vi "Request Synchronous Variant.vi"(6 "Ignore Past Updates? (F)":bool, 7 "Timeout In ms (-1)":i32=-1, 8 "error in (no error)":errorcluster, 9 "Type":variant, 10 "Datum Name":string, 11 "IObserver In":refnum<class "IObserver.lvclass">) -> (0 "error out":errorcluster, 1 "timed out?":bool, 2 "Data":variant, 4 "Publication Time":timestamp)   [LabVIEW 2020, in "IObserver.lvlib" / "IObserver.lvclass"]
doc: "DEPRECATED by Request Synchronous Data.vim"
uses:
  <vilib>/gpm_packages/@cs/mva-core/Source/IObserver/IObserver/IObserver.lvclass
  <vilib>/gpm_packages/@cs/mva-core/Source/IObserver/IObserver/IObserver.lvclass/IObserver.ctl
  <vilib>/gpm_packages/@cs/mva-core/Source/SubscriptionPolicy/OneShotSubscription/OneShotSubscription.lvclass/OneShotSubscription.ctl
  <vilib>/gpm_packages/@cs/transport/Source/Concrete/NotifierTransport/NotifierTransport.lvclass/NotifierTransport.ctl
  <vilib>/gpm_packages/@cs/mva-core/Source/IMediator/SubscriptionRequest/SubscriptionRequest.lvclass/SubscriptionRequest.ctl
  <vilib>/gpm_packages/@cs/mva-core/Source/IMediator/IMediator Messages/Subscribe Msg/Subscribe Msg.lvclass/Subscribe Msg.ctl
  <vilib>/gpm_packages/@cs/actor-framework-messages/Source/RoundTripMessage/RoundTripMessage.lvclass/RoundTripMessage.ctl
  <vilib>/ActorFramework/Message Enqueuer/Message Enqueuer.lvclass/Message Enqueuer.ctl
  <vilib>/gpm_packages/@cs/actor-framework-messages/Source/RoundTripMessage/Return Round-Trip Message.vi
  <vilib>/ActorFramework/Message Enqueuer/Enqueue.vi
  <vilib>/gpm_packages/@cs/transport/Source/Concrete/NotifierTransport/NotifierTransport.lvclass
  C:/Program Files/National Instruments/LabVIEW 2020/vi.lib/gpm_packages/@cs/transport/Source/ITransport/ITransport.lvclass
  <vilib>/gpm_packages/@cs/mva-core/Source/SubscriptionPolicy/OneShotSubscription/OneShotSubscription.lvclass
  C:/Program Files/National Instruments/LabVIEW 2020/vi.lib/gpm_packages/@cs/mva-core/Source/IMediator/ISubscriptionPolicy/ISubscriptionPolicy.lvclass
  <vilib>/gpm_packages/@cs/mva-core/Source/IMediator/IMediator Messages/Subscribe Msg/Subscribe Msg.lvclass
  C:/Program Files/National Instruments/LabVIEW 2020/vi.lib/gpm_packages/@cs/actor-framework-messages/Source/RoundTripMessage/RoundTripMessage.lvclass
  <vilib>/gpm_packages/@cs/actor-framework-messages/Source/RoundTripMessage/RoundTripMessage.lvclass
  C:/Program Files/National Instruments/LabVIEW 2020/vi.lib/ActorFramework/Message/Message.lvclass
  <vilib>/Utility/error.llb/Error Cluster From Error Code.vi
  <vilib>/ActorFramework/Message Priority Queue/Priority Enqueue.vi
  <vilib>/gpm_packages/@cs/mva-core/Source/IMediator/SubscriptionRequest/SubscriptionRequest.lvclass
  <vilib>/gpm_packages/@cs/mva-core/Source/IMediator/ISubscriptionPolicy/ISubscriptionPolicy.lvclass
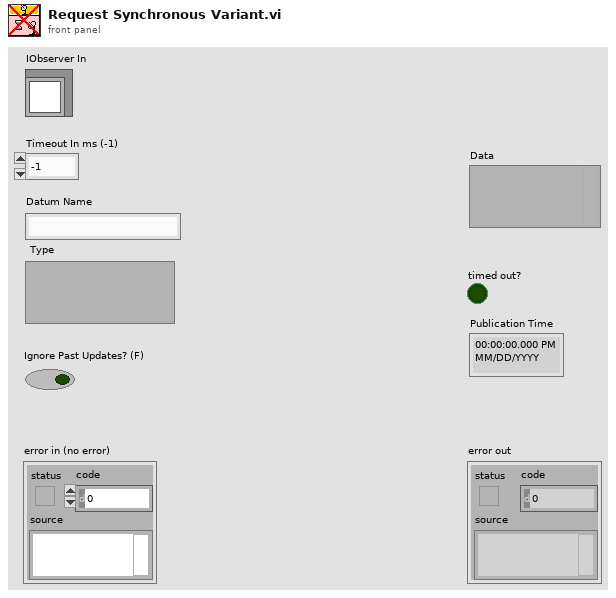
[diagram p1: front panel]
types:
  T1 = typedef "IMediator.lvlib/ISubscriptionPolicy.lvclass/ISubscriptionPolicy Reference.ctl" = refnum<data-value>
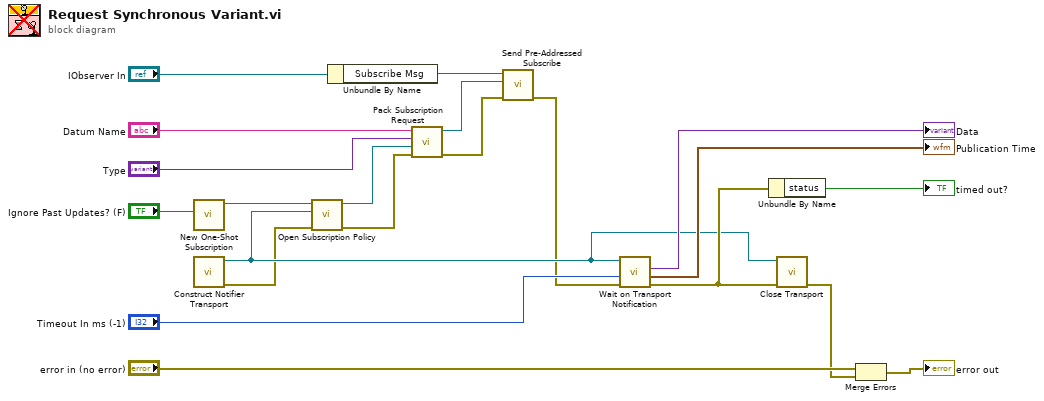
[diagram p0: block diagram]
diagram:
  n1 = call <vilib>:"New One-Shot Subscription.vi"("Ignore Past Updates? (F)"="Ignore Past Updates? (F)") -> ("OneShotSubscription Out"=w18:refnum<class "OneShotSubscription.lvclass">)  [unwired: 10 in]
  n2 = call <vilib>:"Construct Notifier Transport.vi"() -> ("error out"=w4:errorcluster, "NotifierTransport"=w5:refnum<class "NotifierTransport.lvclass">)  [unwired: 10 in]
  n3 = call <vilib>:"Open Subscription Policy.vi"("error in (no error)"=w4, "Transport"=w5, "SubscriptionPolicy"=w18) -> ("error out"=w2:errorcluster, "Subscription Policy"=w6:T1)  [unwired: 7 in]
  n4 = Unbundle By Name("IObserver In") -> ("Subscribe Msg"=w15:refnum<class "Subscribe Msg.lvclass">)
  n5 = call <vilib>:"Pack Subscription Request.vi"("error in (no error)"=w2, "Subscription Policy"=w6, "Type"="Type", "Datum Name"="Datum Name") -> ("error out"=w1:errorcluster, "SubscriptionRequest"=w14:refnum<class "SubscriptionRequest.lvclass">)  [unwired: 6 in]
  n6 = call <vilib>:"Send Pre-Addressed Subscribe.vi"("error in (no error)"=w1, "Subscription Request"=w14, "Subscribe Msg"=w15) -> ("error out"=w3:errorcluster)  [unwired: 8 in]
  n7 = call <vilib>:"Wait on Transport Notification.vi"("error in (no error)"=w3, "Timeout In ms (-1)"="Timeout In ms (-1)", "NotifierTransport"=w5) -> ("error out"=w7:errorcluster, "Publication Time"=→"Publication Time":timestamp, "Data"=→"Data":variant)  [unwired: 6 in]
  n8 = Unbundle By Name(w7) -> ("status"=→"timed out?":bool)
  n9 = call-dynamic "Close Transport.vi"("error in (no error)"=w7, "NotifierTransport"=w5) -> ("error out"=w9:errorcluster)  [unwired: 9 in]
  n10 = Merge Errors("error in (no error)", w9) -> (→"error out":errorcluster)
